vi "FW102C_control.vi"(0 "FW102C in":i32, 1 "Overide pos":i32, 2 "Current Wavelength":dbl, 3 "error in (no error)":errorcluster, 4 "Overide":bool) -> (5 "FW102C out":i32, 6 "Position":i32, 7 "error out":errorcluster)   [LabVIEW 2020]
uses:
  Other_Libraries/Thorlabs_FW102C/Thorlabs_FW102C.lvlib
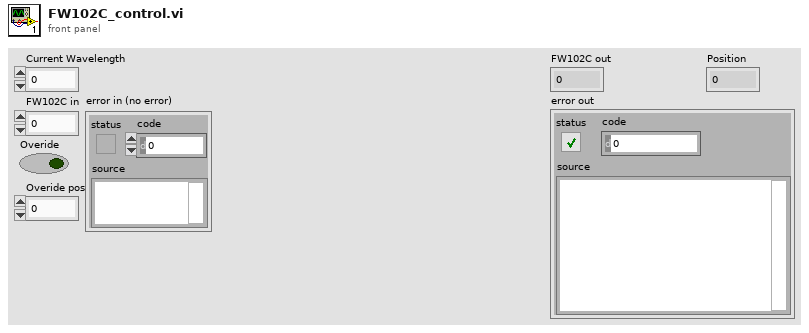
[diagram p1: front panel]
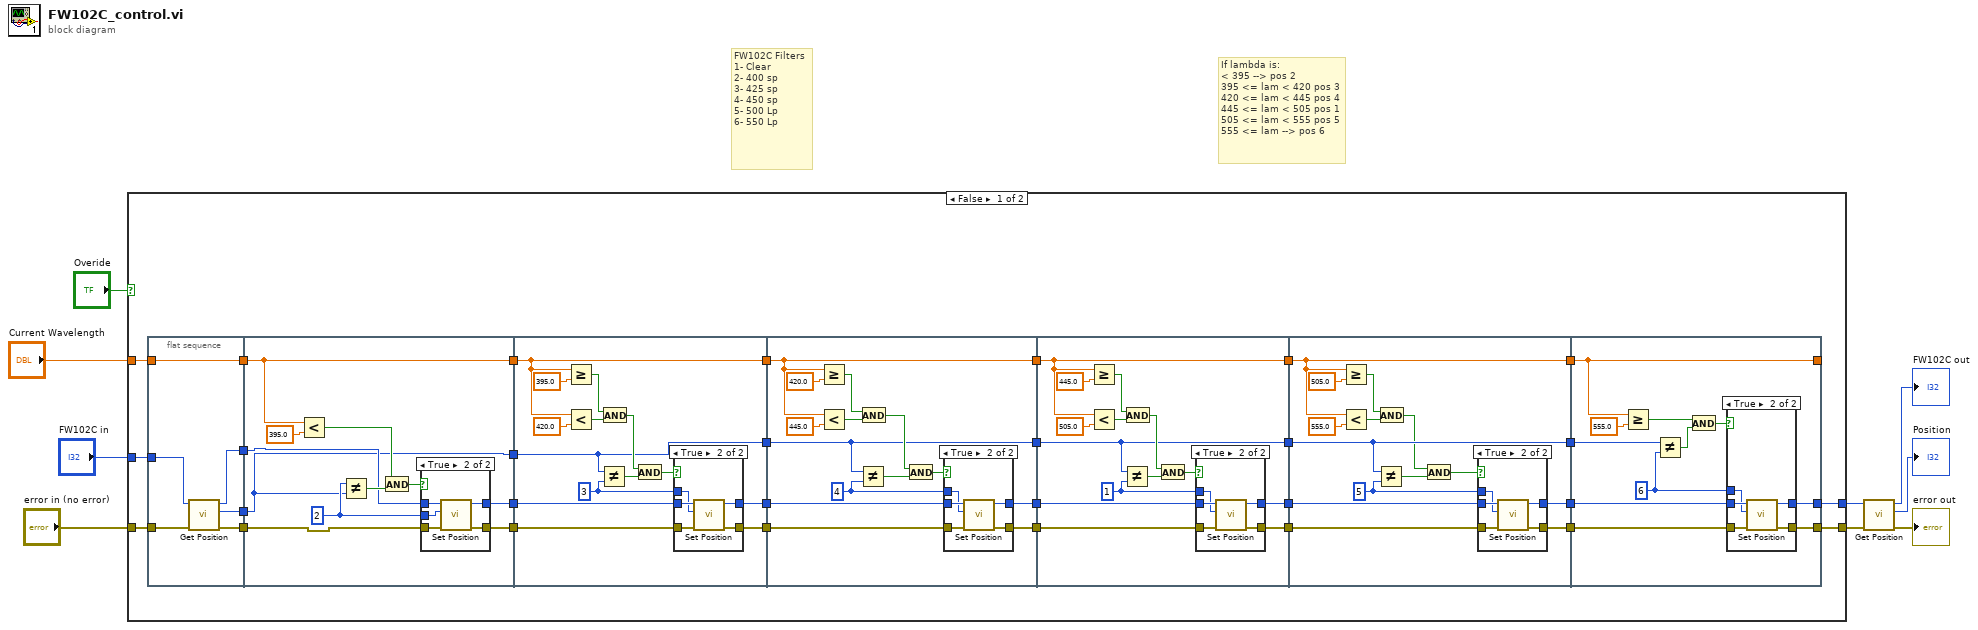
[diagram p0: block diagram]
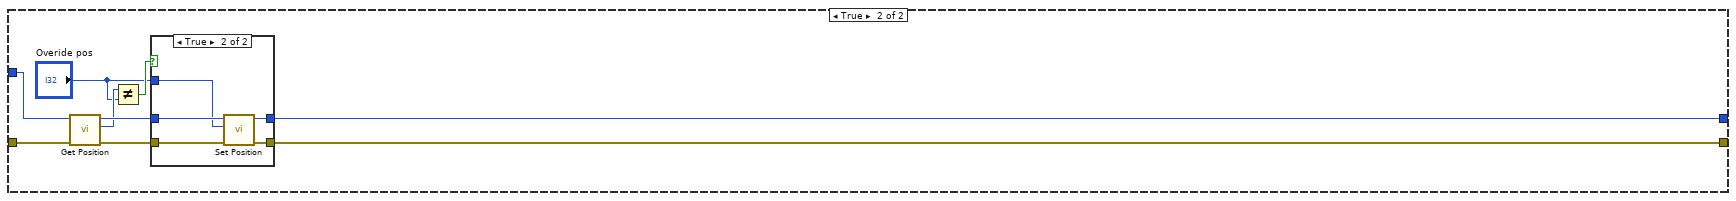
[diagram p8: hidden frame]
diagram:
  # "If lambda is: \n< 395 --> pos 2\n395 <= lam < 420 pos 3\n420 <= lam < 445 pos 4\n445 <= lam < 505 pos 1\n505 <= lam < 555 pos 5\n555 <= lam --> pos 6"
  # "FW102C Filters\n1- Clear\n2- 400 sp\n3- 425 sp\n4- 450 sp \n5- 500 Lp\n6- 550 Lp"
  n1 = case shown="False" "Overide" {
    tunnel: "Current Wavelength" -> [w14 _]
    tunnel: "FW102C in" -> [w13 w172]
    tunnel: "error in (no error)" -> [w12 w173]
    tunnel: [w11 w166] -> w6
    tunnel: [w10 w165] -> w4
    frame False {
      n2 = flat-sequence {
        tunnel: w13 -> [w43]
        tunnel: w14 -> [w44]
        tunnel: [w44] -> w38
        tunnel: [w42] -> w37
        tunnel: [w41] -> w36
        tunnel: w12 -> [w40]
        tunnel: [w39] -> w35
        tunnel: w38 -> [w48]
        tunnel: w37 -> [w47]
        tunnel: w36 -> [w51]
        tunnel: w35 -> [w49]
        tunnel: [w48] -> w34
        tunnel: [w47] -> w33
        tunnel: [w46] -> w32
        tunnel: [w45] -> w31
        tunnel: w34 -> [w66]
        tunnel: w33 -> [w67]
        tunnel: w32 -> [w68]
        tunnel: w31 -> [w69]
        tunnel: [w67] -> w30
        tunnel: [w66] -> w29
        tunnel: [w65] -> w28
        tunnel: [w64] -> w27
        tunnel: w30 -> [w84]
        tunnel: w29 -> [w91]
        tunnel: w28 -> [w89]
        tunnel: [w88] -> w26
        tunnel: [w84] -> w25
        tunnel: [w86] -> w24
        tunnel: w27 -> [w87]
        tunnel: [w91] -> w23
        tunnel: [w111] -> w22
        tunnel: w26 -> [w112]
        tunnel: [w106] -> w21
        tunnel: w25 -> [w106]
        tunnel: [w109] -> w20
        tunnel: w24 -> [w110]
        tunnel: [w113] -> w19
        tunnel: w23 -> [w113]
        tunnel: [w131] -> w18
        tunnel: w22 -> [w132]
        tunnel: [w139] -> w17
        tunnel: w21 -> [w139]
        tunnel: [w129] -> w16
        tunnel: w20 -> [w130]
        tunnel: [w135] -> w15
        tunnel: w19 -> [w135]
        tunnel: [w153] -> w11
        tunnel: w18 -> [w154]
        tunnel: w17 -> [w157]
        tunnel: [w151] -> w10
        tunnel: w16 -> [w152]
        tunnel: [w147] -> _
        tunnel: w15 -> [w147]
        frame #0 {
          n3 = call "Get Position.vi"("error in (no error)"=w40, "FW102C in"=w43) -> ("error out"=w39:errorcluster, "Position"=w42:i32, "FW102C out"=w41:i32)  [unwired: 7 in]
        }
        frame #1 {
          w50 = 2 ("x")
          n4 = Less?(x=w48, y=395.0) -> (x < y?=w54:bool)
          n5 = Not Equal?(x=w50, y=w47) -> (x != y?=w53:bool)
          n6 = And(x=w54, y=w53) -> (x .and. y?=w52:bool)
          n7 = case shown="True" w52 {
            tunnel: w51 -> [w57 w62]
            tunnel: w50 -> [_ w61]
            tunnel: [w57 w60] -> w46
            tunnel: w49 -> [w56 w59]
            tunnel: [w56 w58] -> w45
            frame False {
            }
            frame True {
              n8 = call "Set Position.vi"("error in (no error)"=w59, "Position"=w61, "FW102C in"=w62) -> ("error out"=w58:errorcluster, "FW102C out"=w60:i32)  [unwired: 7 in]
            }
          }
        }
        frame #2 {
          w63 = 3 ("y")
          n9 = Greater Or Equal?(x=w66, y=395.0) -> (x >= y?=w74:bool)
          n10 = Less?(x=w66, y=420.0) -> (x < y?=w73:bool)
          n11 = Not Equal?(x=w67, y=w63) -> (x != y?=w76:bool)
          n12 = And(x=w74, y=w73) -> (x .and. y?=w71:bool)
          n13 = And(x=w71, y=w76) -> (x .and. y?=w70:bool)
          n14 = case shown="True" w70 {
            tunnel: w68 -> [w78 w83]
            tunnel: w63 -> [_ w82]
            tunnel: [w78 w81] -> w64
            tunnel: w69 -> [w77 w80]
            tunnel: [w77 w79] -> w65
            frame False {
            }
            frame True {
              n15 = call "Set Position.vi"("error in (no error)"=w80, "Position"=w82, "FW102C in"=w83) -> ("error out"=w79:errorcluster, "FW102C out"=w81:i32)  [unwired: 7 in]
            }
          }
        }
        frame #3 {
          w85 = 4 ("y")
          n16 = Greater Or Equal?(x=w91, y=420.0) -> (x >= y?=w95:bool)
          n17 = Less?(x=w91, y=445.0) -> (x < y?=w94:bool)
          n18 = Not Equal?(x=w84, y=w85) -> (x != y?=w97:bool)
          n19 = And(x=w95, y=w94) -> (x .and. y?=w92:bool)
          n20 = And(x=w92, y=w97) -> (x .and. y?=w90:bool)
          n21 = case shown="True" w90 {
            tunnel: w87 -> [w99 w104]
            tunnel: w85 -> [_ w103]
            tunnel: [w99 w102] -> w86
            tunnel: w89 -> [w98 w101]
            tunnel: [w98 w100] -> w88
            frame False {
            }
            frame True {
              n22 = call "Set Position.vi"("error in (no error)"=w101, "Position"=w103, "FW102C in"=w104) -> ("error out"=w100:errorcluster, "FW102C out"=w102:i32)  [unwired: 7 in]
            }
          }
        }
        frame #4 {
          w108 = 1 ("y")
          n23 = Greater Or Equal?(x=w113, y=445.0) -> (x >= y?=w114:bool)
          n24 = Less?(x=w113, y=505.0) -> (x < y?=w117:bool)
          n25 = Not Equal?(x=w106, y=w108) -> (x != y?=w107:bool)
          n26 = And(x=w114, y=w117) -> (x .and. y?=w115:bool)
          n27 = And(x=w115, y=w107) -> (x .and. y?=w105:bool)
          n28 = case shown="True" w105 {
            tunnel: w110 -> [w120 w125]
            tunnel: w108 -> [_ w124]
            tunnel: [w120 w123] -> w109
            tunnel: w112 -> [w119 w122]
            tunnel: [w119 w121] -> w111
            frame False {
            }
            frame True {
              n29 = call "Set Position.vi"("error in (no error)"=w122, "Position"=w124, "FW102C in"=w125) -> ("error out"=w121:errorcluster, "FW102C out"=w123:i32)  [unwired: 7 in]
            }
          }
        }
        frame #5 {
          w128 = 5 ("y")
          n30 = Greater Or Equal?(x=w135, y=505.0) -> (x >= y?=w134:bool)
          n31 = Less?(x=w135, y=555.0) -> (x < y?=w137:bool)
          n32 = Not Equal?(x=w139, y=w128) -> (x != y?=w133:bool)
          n33 = And(x=w134, y=w137) -> (x .and. y?=w136:bool)
          n34 = And(x=w136, y=w133) -> (x .and. y?=w127:bool)
          n35 = case shown="True" w127 {
            tunnel: w130 -> [w141 w146]
            tunnel: w128 -> [_ w145]
            tunnel: [w141 w144] -> w129
            tunnel: w132 -> [w140 w143]
            tunnel: [w140 w142] -> w131
            frame False {
            }
            frame True {
              n36 = call "Set Position.vi"("error in (no error)"=w143, "Position"=w145, "FW102C in"=w146) -> ("error out"=w142:errorcluster, "FW102C out"=w144:i32)  [unwired: 7 in]
            }
          }
        }
        frame #6 {
          w155 = 6 ("y")
          n37 = Greater Or Equal?(x=w147, y=555.0) -> (x >= y?=w148:bool)
          n38 = Not Equal?(x=w157, y=w155) -> (x != y?=w150:bool)
          n39 = And(x=w148, y=w150) -> (x .and. y?=w149:bool)
          n40 = case shown="True" w149 {
            tunnel: w152 -> [w159 w164]
            tunnel: w155 -> [_ w163]
            tunnel: [w159 w162] -> w151
            tunnel: w154 -> [w158 w161]
            tunnel: [w158 w160] -> w153
            frame False {
            }
            frame True {
              n41 = call "Set Position.vi"("error in (no error)"=w161, "Position"=w163, "FW102C in"=w164) -> ("error out"=w160:errorcluster, "FW102C out"=w162:i32)  [unwired: 7 in]
            }
          }
        }
      }
    }
    frame True {
      n42 = call "Get Position.vi"("error in (no error)"=w173, "FW102C in"=w172) -> ("error out"=w167:errorcluster, "Position"=w170:i32, "FW102C out"=w171:i32)  [unwired: 7 in]
      n43 = Not Equal?(x=w170, y="Overide pos") -> (x != y?=w169:bool)
      n44 = case shown="True" w169 {
        tunnel: w171 -> [w175 w180]
        tunnel: "Overide pos" -> [_ w179]
        tunnel: w167 -> [w174 w178]
        tunnel: [w174 w177] -> w166
        tunnel: [w175 w176] -> w165
        frame False {
        }
        frame True {
          n45 = call "Set Position.vi"("error in (no error)"=w178, "Position"=w179, "FW102C in"=w180) -> ("error out"=w177:errorcluster, "FW102C out"=w176:i32)  [unwired: 7 in]
        }
      }
    }
  }
  n46 = call "Get Position.vi"("error in (no error)"=w6, "FW102C in"=w4) -> ("error out"=→"error out":errorcluster, "Position"=→"Position":i32, "FW102C out"=→"FW102C out":i32)  [unwired: 7 in]
